vi "divide_beta.vi"(0 "INPUT":T2) -> (1 "OVERFLOW":bool, 2 "OUTPUT":T1)   [LabVIEW 2013]
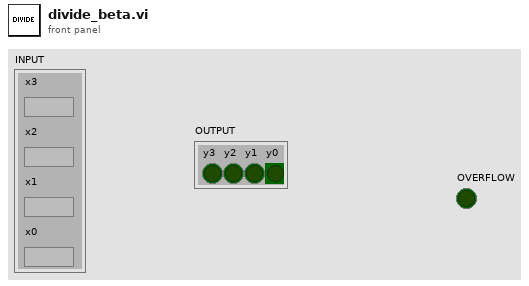
[diagram p1: front panel]
types:
  T1 = cluster{"y3":bool, "y2":bool, "y1":bool, "y0":bool}
  T2 = cluster{"x3":bool, "x2":bool, "x1":bool, "x0":bool}
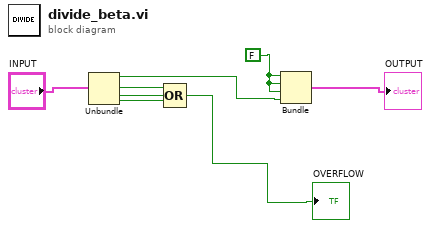
[diagram p0: block diagram]
diagram:
  w1 = FALSE
  n1 = Unbundle("INPUT") -> ("x3"=w2:bool, "x2"=w5:bool, "x1"=w4:bool, "x0"=w3:bool)
  n2 = Compound Arithmetic op=OR(w5, w4, w3) -> (→"OVERFLOW":bool)
  n3 = Bundle(w1, w1, w1, "x3"=w2) -> (→"OUTPUT":cluster{bool, bool, bool, "x3":bool})  [unwired: 1 in]
